vi "Dequeue.vi"(11 "Base Queue in":refnum<class "Base Queue.lvclass">) -> (2 "Msg Strategy":refnum<class "Msg Strategy.lvclass">, 3 "Base Queue out":refnum<class "Base Queue.lvclass">)   [LabVIEW 2021, in "jettl.lvlib" / "Base Queue.lvlib" / "Base Queue.lvclass"]
uses:
  Base Queue.lvclass
  Base Queue.lvclass/Base Queue.ctl
  Msg Type Strategy/Queue Msg Type Strategy/Queue Msg Type Strategy.lvclass
  Addresses/Addresses.lvlib
  Msg Strategy/Msg Strategy.lvclass
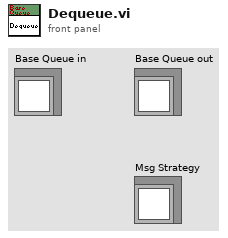
[diagram p1: front panel]
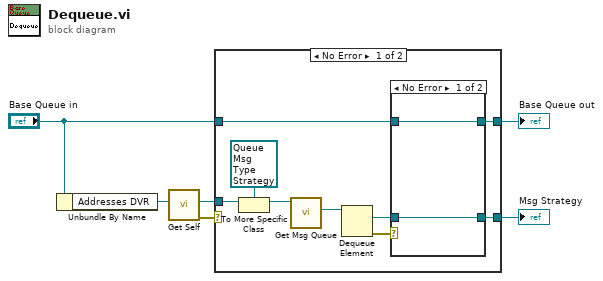
[diagram p0: block diagram]
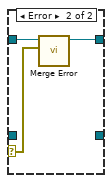
[diagram p2: hidden frame]
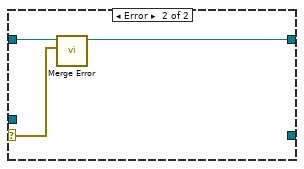
[diagram p3: hidden frame]
diagram:
  n1 = Unbundle By Name("Base Queue in") -> ("Addresses DVR"=w5:refnum<data-value>)
  n2 = call "Get Self.vi"("Addresses DVR"=w5) -> ("error out"=w1:errorcluster, "Self"=w3:refnum<class "Msg Type Strategy.lvclass">)  [unwired: 9 in]
  n3 = case shown="No Error" w1 {
    selector: w1 -> [_ w21]
    tunnel: [w15 w23] -> w6
    tunnel: "Base Queue in" -> [w14 w22]
    tunnel: w3 -> [w13 _]
    tunnel: [w8 _] -> w2
    frame No Error {
      n4 = To More Specific Class(target class=refnum<class "Queue Msg Type Strategy.lvclass"> refnum ("jettl.lvlib:Msg Type Strategy.lvlib:Queue Msg Type Strategy.lvclass"), reference=w13) -> (specific class reference=w12:refnum<class "Queue Msg Type Strategy.lvclass">)  [unwired: 1 in, 1 out]
      n5 = call "Get Msg Queue.vi"("Queue Msg Type Strategy in"=w12) -> ("Msg Queue"=w10:refnum<queue>)  [unwired: 10 in]
      n6 = Dequeue Element(queue=w10) -> (element=w7:refnum<class "Msg Strategy.lvclass">, error out=w9:errorcluster)  [unwired: 2 in, 2 out]
      n7 = case shown="No Error" w9 {
        selector: w9 -> [_ w18]
        tunnel: [w16 w20] -> w15
        tunnel: w14 -> [w16 w19]
        tunnel: [w17 _] -> w8
        tunnel: w7 -> [w17 _]
        frame No Error {
        }
        frame Error {
          n8 = call-dynamic "Merge Error.vi"("Error"=w18, "Base Queue in"=w19) -> ("Base Queue out"=w20:refnum<class "Base Queue.lvclass">)  [unwired: 9 in]
        }
      }
    }
    frame Error {
      n9 = call-dynamic "Merge Error.vi"("Error"=w21, "Base Queue in"=w22) -> ("Base Queue out"=w23:refnum<class "Base Queue.lvclass">)  [unwired: 9 in]
    }
  }
  "Base Queue out" <- w6
  "Msg Strategy" <- w2
